vi "globalSetUp.vi"(8 "error in":errorcluster, 11 "Single Board Loopback in":refnum<class "Single Board Loopback.lvclass">) -> (0 "error out":errorcluster, 3 "Single Board Loopback out":refnum<class "Single Board Loopback.lvclass">)   [LabVIEW 2020, in "Single Board Loopback.lvclass"]
uses:
  Single Board Loopback.lvclass
  <vilib>/NI/VeriStand Custom Device Testing Tools/VeriStandTestUtilities/VeriStandTestUtilities.lvlib
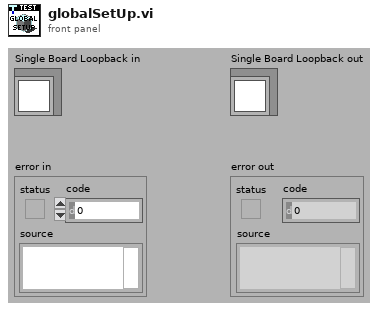
[diagram p1: front panel]
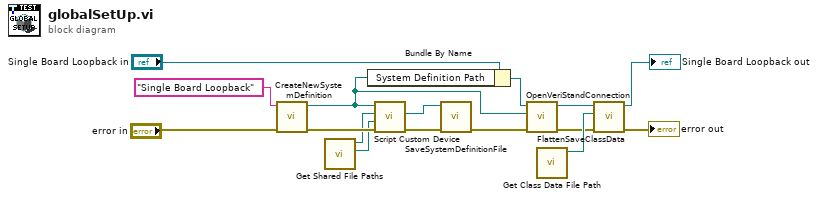
[diagram p0: block diagram]
diagram:
  n1 = call <vilib>:"CreateNewSystemDefinition.vi"("error in"="error in", "System Definition Name"="Single Board Loopback" ("Channel")) -> ("error out"=w13:errorcluster, "System Definition Path"=w4:path)  [unwired: 8 in]
  n2 = call "Get Shared File Paths.vi"() -> ("Hardware File"=w1:path, "Parameters File"=w2:path)  [unwired: 10 in]
  n3 = Bundle By Name(cluster="Single Board Loopback in", "System Definition Path"=w4) -> (w6:refnum<class "Single Board Loopback.lvclass">)
  n4 = call "Script Custom Device.vi"("error in"=w13, "Hardware Configuration File Path"=w1, "Parameters Configuration File Path"=w2, "System Definition File Path In"=w4) -> ("error out"=w16:errorcluster, "System Definition Reference"=w11:refnum<k24>)  [unwired: 4 in, 2 out]
  n5 = call <vilib>:"SaveSystemDefinitionFile.vi"("error in (no error)"=w16, "System Definition Reference in"=w11) -> ("error out"=w12:errorcluster)  [unwired: 8 in, 1 out]
  n6 = call-dynamic "OpenVeriStandConnection.vi"("error in (no error)"=w12, "System Definition File"=w4, "VeriStand Test Case in"=w6) -> ("error out"=w7:errorcluster, "VeriStand Test Case out"=w3:refnum<class "Single Board Loopback.lvclass">)  [unwired: 6 in, 1 out]
  n7 = call "Get Class Data File Path.vi"() -> ("Class Data File Path"=w8:path)  [unwired: 11 in]
  n8 = call-dynamic "FlattenSaveClassData.vi"("error in"=w7, "Class Data File Path"=w8, "VeriStandTestCase in"=w3) -> ("error out"=→"error out":errorcluster, "VeriStandTestCase out"=→"Single Board Loopback out":refnum<class "Single Board Loopback.lvclass">)  [unwired: 7 in]
